vi "SnapAndParthing2.vi"(10 "Result Arr":T1(array[cluster]), 11 "Vision&Robot":refnum<vi>) -> (3 "Name":string[](array[string]))   [LabVIEW 2019]
uses:
  VisionSet/System/iVision/Controls/Parameter.ctl
  6eb8f04b-a15a-4811-94d3-d4eebb3499ca.vi
  <vilib>/Array/Sort 2D Array - Pop Stack.vi
  <vilib>/Array/Sort 2D Array - Push Stack.vi
  6eb8f04b-a15a-4811-94d3-d4eebb3499ca.vi/becce5ee-4515-45bf-9efc-18b6bc445c2a.vi
  6eb8f04b-a15a-4811-94d3-d4eebb3499ca.vi/625cd210-0173-46f9-a6ca-1fcbc6d231a4.vi
panel:
  out "sorted 2D array":dbl[][](array[numeric])
  # "P_X_1"
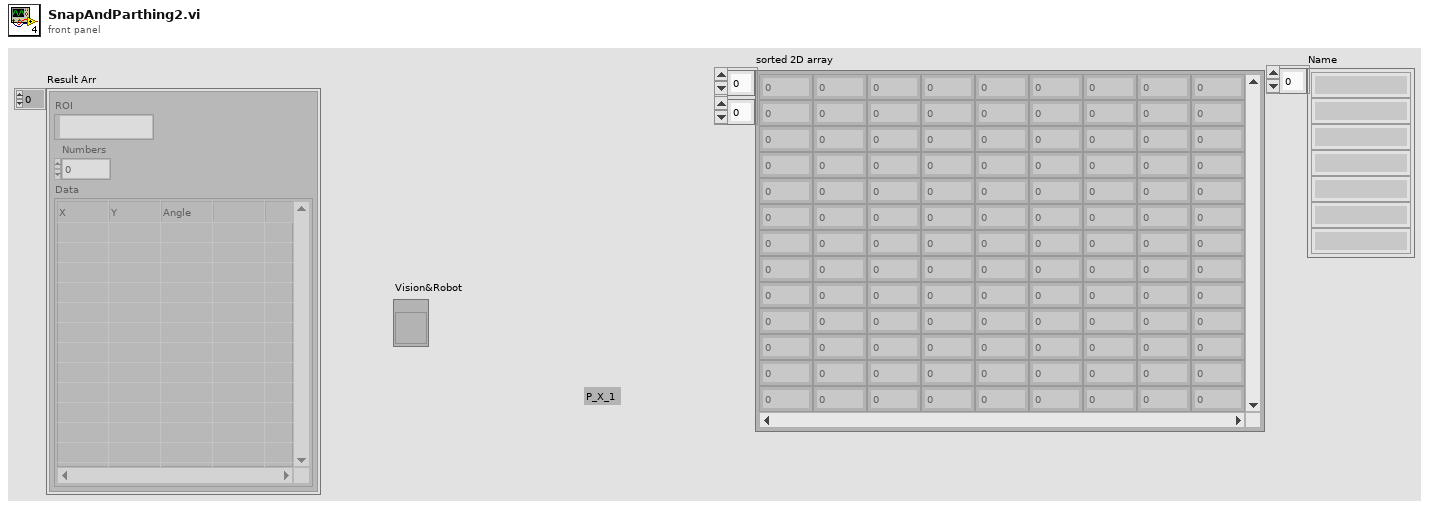
[diagram p1: front panel]
types:
  T1 = cluster{"ROI":string, "Numbers":i32, "Data":string[][]}[]
  T2 = typedef "Parameter.ctl" = enum16{"Initialize", "Write", "Read", "WriteAll", "Save", "Load"}
  T3 = typedef "ParameterData.ctl" = cluster{"Rotate Angle":dbl, "Rotate?":bool, "Calibration File Path":string, "Cal?":bool}
  T4 = cluster{"VisionPoint":cluster{"X":dbl, "Y":dbl}, "RobotPoint":cluster{"X":dbl, "Y":dbl, "U":dbl}}[]
  T5 = cluster{"VisionPoint":cluster{"X":dbl, "Y":dbl}, "RobotPoint":cluster{"X":dbl, "Y":dbl, "U":dbl}}
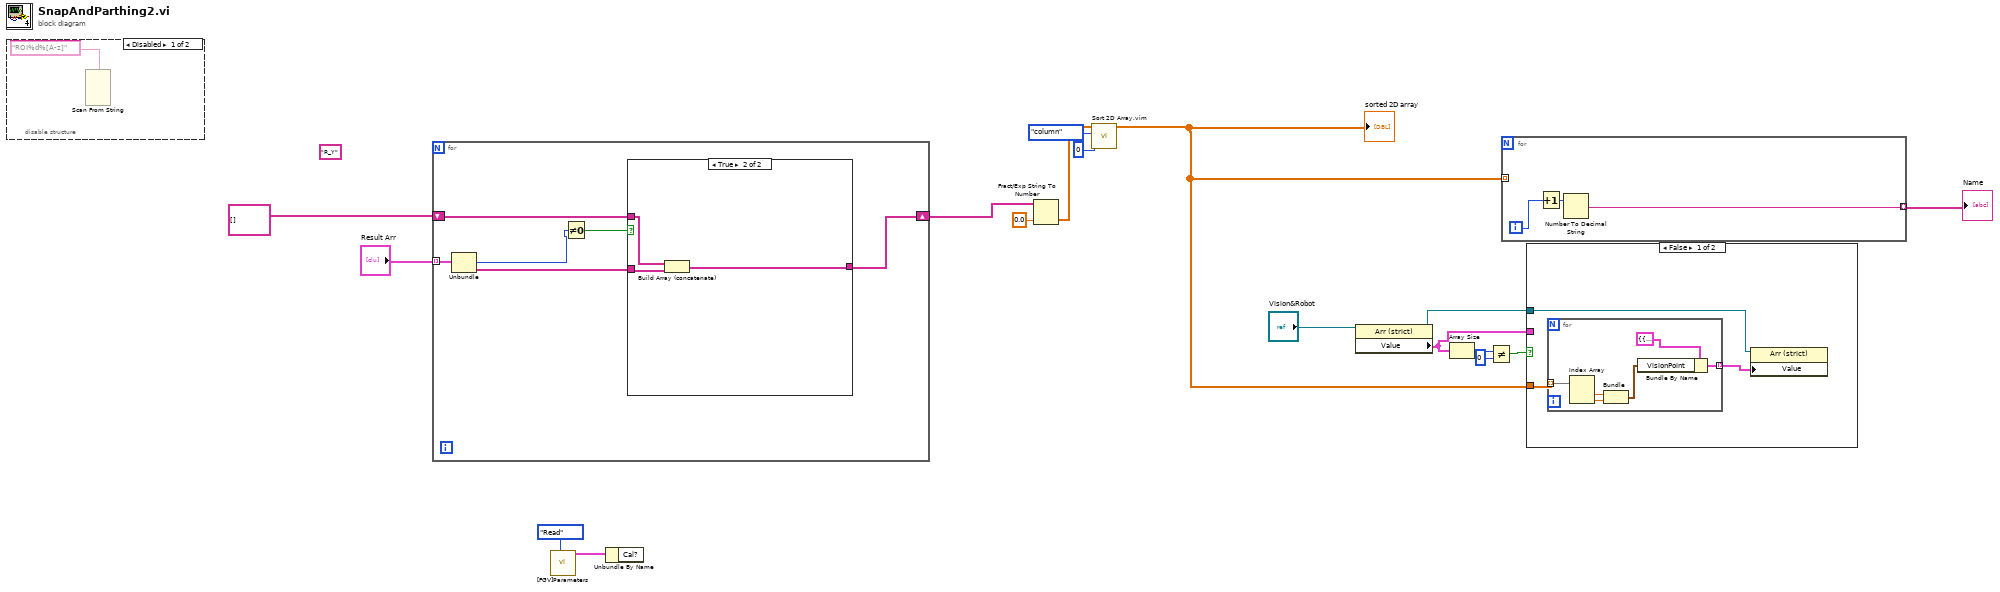
[diagram p0: block diagram]
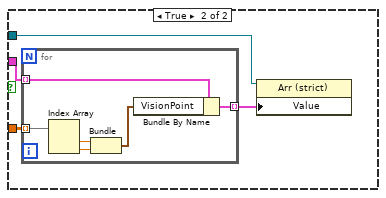
[diagram p2: hidden frame]
diagram:
  (unwired) "R_Y"
  n1 = disable-structure shown="Disabled" {
    frame Disabled {
      n2 = Scan From String(format string="ROI%d%[A-z]") -> ()  [unwired: 7 in, 3 out]
    }
    frame Enabled {
    }
  }
  n3 = for {
    tunnel: "Result Arr" -> [w24] mode=indexing
    shift-right: [w20] -> w12
    shift-left: string[][] [] -> [w19]
    n4 = Unbundle(w24) -> ("Numbers"=w23:i32, "Data"=w21:string[][])  [unwired: 1 out]
    n5 = Not Equal To 0?(x=w23) -> (x != 0?=w22:bool)
    n6 = case shown="True" w22 {
      tunnel: w21 -> [_ w28]
      tunnel: [w25 w27] -> w20
      tunnel: w19 -> [w25 w26]
      frame False {
      }
      frame True {
        n7 = Build Array (concatenate)(w26, w28) -> (w27:string[][])
      }
    }
  }
  n8 = call "[FGV]Parameters.vi"("Parameter"=Parameter."Read") -> ("ParameterData Out"=w17:T3)  [unwired: 9 in, 1 out]
  n9 = Unbundle By Name(w17) -> ()  [unwired: 1 out]
  n10 = Fract/Exp String To Number(string=w12, default (0 dbl)=0.0 ("default (0 DBL)")) -> (number=w11:dbl[][])  [unwired: 2 in, 1 out]
  n11 = call "Sort 2D Array.vim"("index"=0, "dimension to index (column)"=enum16{"column", "row"}."column", "2D array"=w11) -> ("sorted 2D array"=w2:dbl[][])  [unwired: 7 in, 1 out]
  "sorted 2D array" <- w2
  n12 = property class="Arr (strict)"(reference="Vision&Robot") -> (reference out=w8:refnum<vi>, "Value"=w4:T4)  [unwired: 1 in, 1 out]
  n13 = Array Size(array=w4) -> (size(s)=w6:i32)
  n14 = Not Equal?(x=w6, y=0) -> (x != y?=w5:bool)
  n15 = for {
    tunnel: w2 -> [_] mode=indexing
    tunnel: [w29] -> w1 mode=indexing
    i -> [w31]
    n16 = Increment(x=w31) -> (x+1=w30:i32)
    n17 = Number To Decimal String(number=w30) -> (decimal integer string=w29:string)  [unwired: 1 in]
  }
  "Name" <- w1
  n18 = case shown="False" w5 {
    tunnel: w8 -> [w34 w44]
    tunnel: w2 -> [w32 w42]
    tunnel: w4 -> [_ w41]
    frame False {
      n19 = for {
        tunnel: [w40] -> w33 mode=indexing
        tunnel: w32 -> [w36] mode=indexing
        n20 = Index Array(array=w36) -> (element #1=w39:dbl, element #2=w38:dbl)  [unwired: 2 in]
        n21 = Bundle(w39, w38) -> (w35:cluster{dbl, dbl})  [unwired: 1 in]
        n22 = Bundle By Name(cluster=T5 {"VisionPoint"={"X"=0.0, "Y"=0.0}, "RobotPoint"={"X"=0.0, "Y"=0.0, "U"=0.0}} ("Data"), "VisionPoint"=w35) -> (w40:T5)
      }
      n23 = property class="Arr (strict)"(reference=w34, "Value"=w33) -> ()  [unwired: 1 in, 2 out]
    }
    frame True {
      n24 = for {
        tunnel: w41 -> [w50] mode=indexing
        tunnel: [w49] -> w43 mode=indexing
        tunnel: w42 -> [w46] mode=indexing
        n25 = Index Array(array=w46) -> (element #1=w48:dbl, element #2=w47:dbl)  [unwired: 2 in]
        n26 = Bundle(w48, w47) -> (w45:cluster{dbl, dbl})  [unwired: 1 in]
        n27 = Bundle By Name(cluster=w50, "VisionPoint"=w45) -> (w49:T5)
      }
      n28 = property class="Arr (strict)"(reference=w44, "Value"=w43) -> ()  [unwired: 1 in, 2 out]
    }
  }
